vi "Test-Streaming.vi"() -> ()   [LabVIEW 2020]
uses:
  g_industrial_cam/Camera/Camera.lvclass
  g_industrial_cam/Buffer/Buffer.lvclass
  <vilib>/picture/picture.llb/Draw 8-Bit Pixmap.vi
  g_industrial_cam/Device Enumeration.ctl
panel:
  out "Trigger Source":string
  out "Streaming":bool
  out "Stream Restart Error":errorcluster
  in  "Stop Stream":bool
  in  "Start Stream":bool
  out "Timeout":bool
  out "Devices":T1[](array[typedef])
  in  "Picture Zoom Factor":sgl
  out "2D Picture":picture
  out "Snap Shot Count":i32
  in  "stop":bool
  out "error out":errorcluster
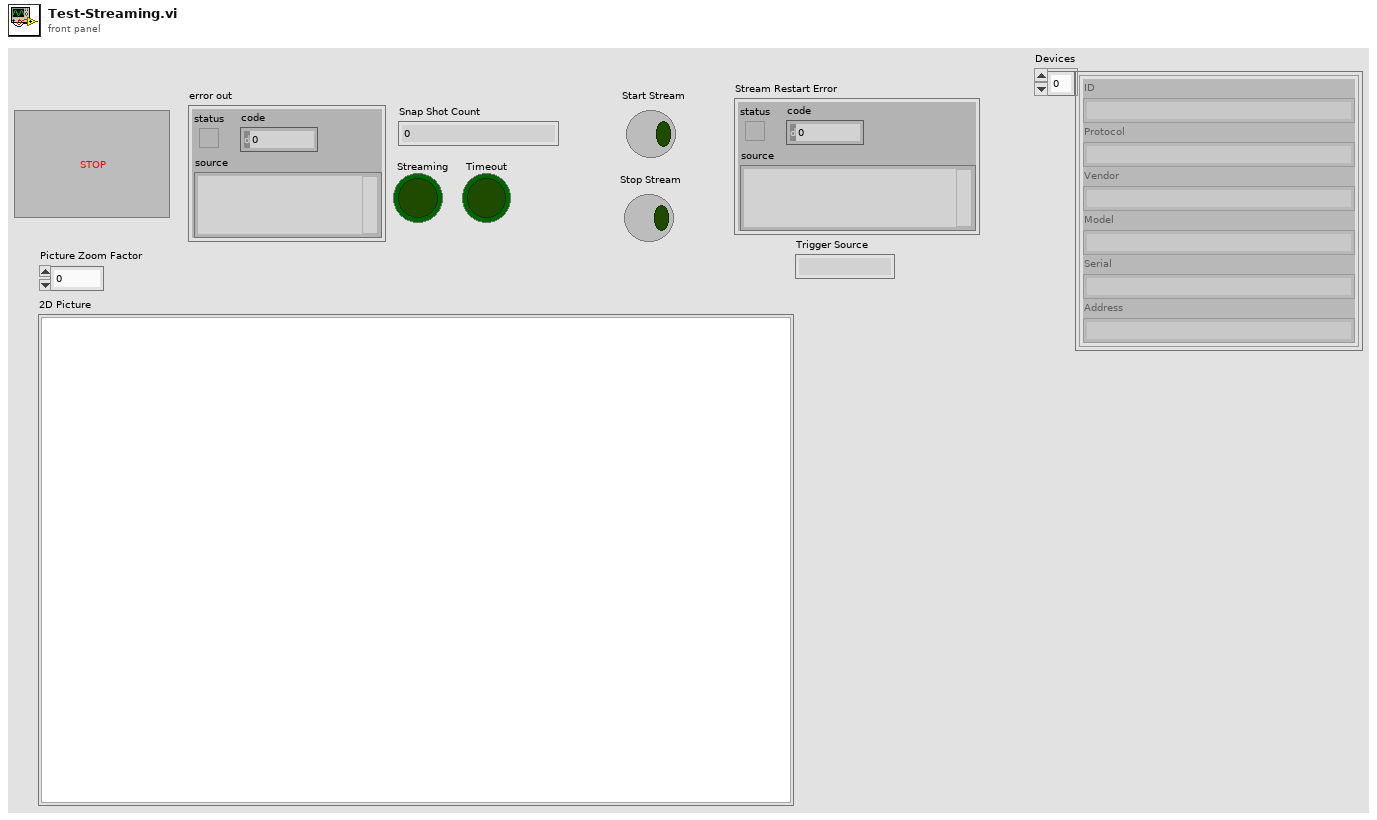
[diagram p1: front panel]
types:
  T1 = typedef "Device Enumeration.ctl" = cluster{"ID":string, "Protocol":string, "Vendor":string, "Model":string, "Serial":string, "Address":string}
  T2 = typedef "Buffer.lvclass/Image Size.ctl" = cluster{"Width":u16, "Height":u16}
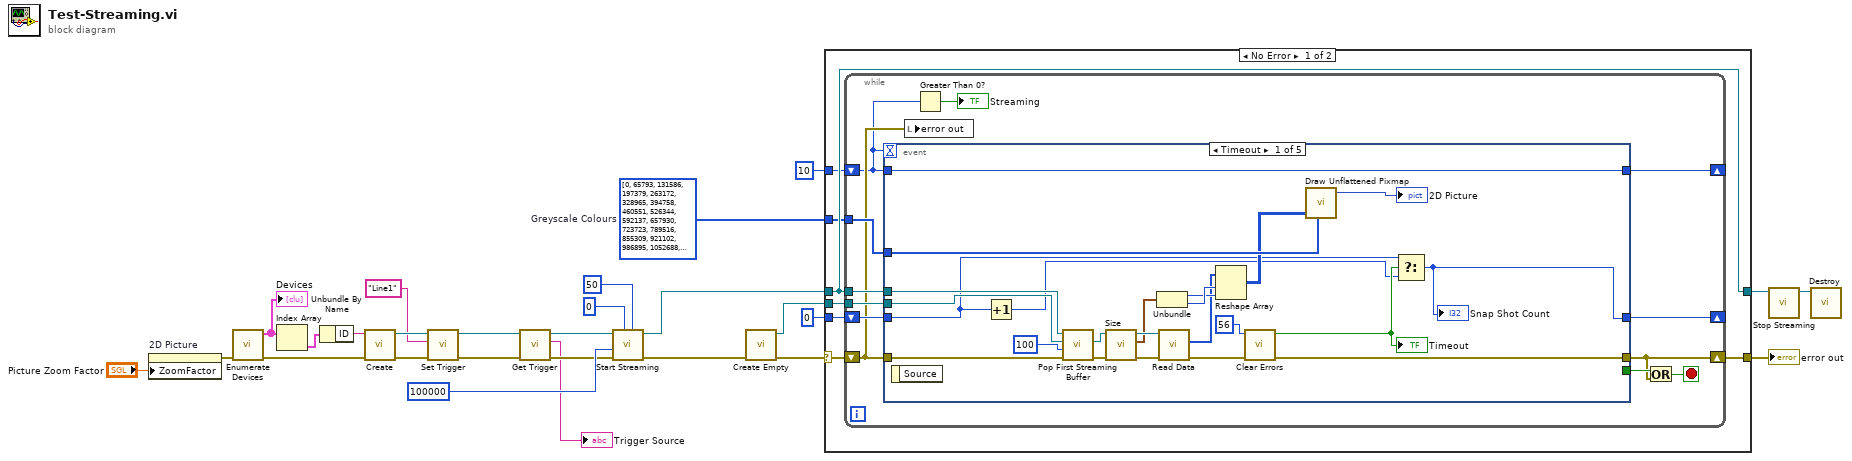
[diagram p0: block diagram]
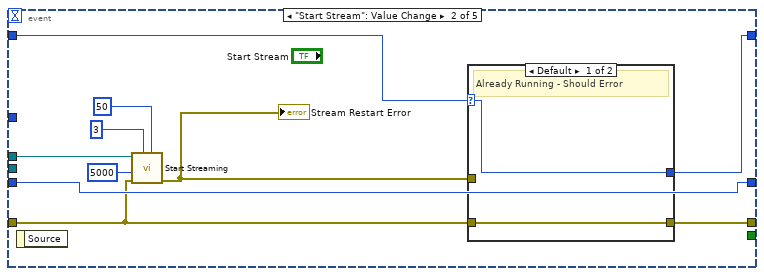
[diagram p2: hidden frame]
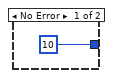
[diagram p4: hidden frame]
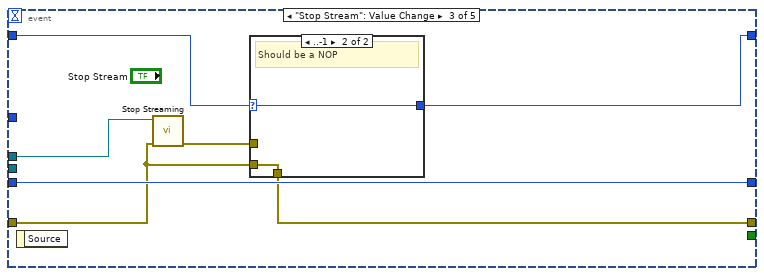
[diagram p5: hidden frame]
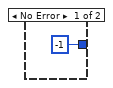
[diagram p7: hidden frame]
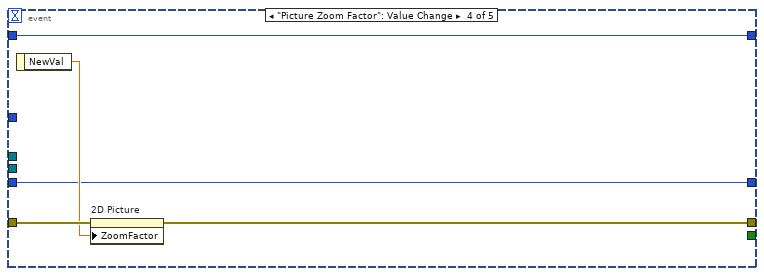
[diagram p8: hidden frame]
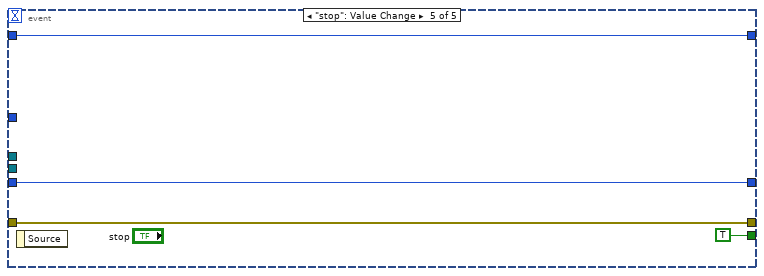
[diagram p9: hidden frame]
diagram:
  w21 = u32[] [0, 65793, 131586, 197379, 263172, 328965, 394758, 460551, 526344, 592137, 657930, 723723, 789516, 855309, 921102, 986895, 1052688, 1118481, 1184274, 1250067, 1315860, 1381653, 1447446, 1513239, 1579032, 1644825, 1710618, 1776411, 1842204, 1907997, 1973790, 2039583, 2105376, 2171169, 2236962, 2302755, 2368548, 2434341, 2500134, 2565927, 2631720, 2697513, 2763306, 2829099, 2894892, 2960685, 3026478, 3092271, 3158064, 3223857, 3289650, 3355443, 3421236, 3487029, 3552822, 3618615, 3684408, 3750201, 3815994, 3881787, 3947580, 4013373, 4079166, 4144959, 4210752, 4276545, 4342338, 4408131, 4473924, 4539717, 4605510, 4671303, 4737096, 4802889, 4868682, 4934475, 5000268, 5066061, 5131854, 5197647, 5263440, 5329233, 5395026, 5460819, 5526612, 5592405, 5658198, 5723991, 5789784, 5855577, 5921370, 5987163, 6052956, 6118749, 6184542, 6250335, 6316128, 6381921, 6447714, 6513507, 6579300, 6645093, 6710886, 6776679, 6842472, 6908265, 6974058, 7039851, 7105644, 7171437, 7237230, 7303023, 7368816, 7434609, 7500402, 7566195, 7631988, 7697781, 7763574, 7829367, 7895160, 7960953, 8026746, 8092539, 8158332, 8224125, 8289918, 8355711, 8421504, 8487297, 8553090, 8618883, 8684676, 8750469, 8816262, 8882055, 8947848, 9013641, 9079434, 9145227, 9211020, 9276813, 9342606, 9408399, 9474192, 9539985, 9605778, 9671571, 9737364, 9803157, 9868950, 9934743, 10000536, 10066329, 10132122, 10197915, 10263708, 10329501, 10395294, 10461087, 10526880, 10592673, 10658466, 10724259, 10790052, 10855845, 10921638, 10987431, 11053224, 11119017, 11184810, 11250603, 11316396, 11382189, 11447982, 11513775, 11579568, 11645361, 11711154, 11776947, 11842740, 11908533, 11974326, 12040119, 12105912, 12171705, 12237498, 12303291, 12369084, 12434877, 12500670, 12566463, 12632256, 12698049, 12763842, 12829635, 12895428, 12961221, 13027014, 13092807, 13158600, 13224393, 13290186, 13355979, 13421772, 13487565, 13553358, 13619151, 13684944, 13750737, 13816530, 13882323, 13948116, 14013909, 14079702, 14145495, 14211288, 14277081, 14342874, 14408667, 14474460, 14540253, 14606046, 14671839, 14737632, 14803425, 14869218, 14935011, 15000804, 15066597, 15132390, 15198183, 15263976, 15329769, 15395562, 15461355, 15527148, 15592941, 15658734, 15724527, 15790320, 15856113, 15921906, 15987699, 16053492, 16119285, 16185078, 16250871, 16316664, 16382457, 16448250, 16514043, 16579836, 16645629, 16711422, 16777215]  # Greyscale Colours
  n1 = property on="2D Picture" class="Pict"("ZoomFactor"="Picture Zoom Factor") -> (error out=w20:errorcluster)  [unwired: 2 in, 1 out]
  n2 = call "Enumerate Devices.vi"("error in (no error)"=w20) -> ("error out"=w25:errorcluster, "Devices"=w27:T1[])  [unwired: 9 in]
  "Devices" <- w27
  n3 = Index Array(array=w27) -> (element=w26:T1)  [unwired: 1 in]
  n4 = Unbundle By Name(w26) -> ("ID"=w24:string)
  n5 = call "Create.vi"("error in (no error)"=w25, "Identifier (ID, IP etc)"=w24) -> ("error out"=w23:errorcluster, "Camera"=w6:refnum<class "Camera.lvclass">)  [unwired: 8 in]
  n6 = call "Set Trigger.vi"("error in (no error)"=w23, "Source"="Line1", "Camera in"=w6) -> ("error out"=w7:errorcluster, "Camera"=w3:refnum<class "Camera.lvclass">)  [unwired: 7 in]
  n7 = call "Get Trigger.vi"("error in (no error)"=w7, "Camera in"=w3) -> ("error out"=w4:errorcluster, "Trigger Source"=→"Trigger Source":string, "Camera"=w2:refnum<class "Camera.lvclass">)  [unwired: 7 in]
  n8 = call "Start Streaming.vi"("Max Sequential Frame-Errors (Default: -1)"=50 ("Max Sequential Errors (Default: -1)"), "Additional Buffers (Default: 3)"=u16 0 ("Additional Buffers (3)"), "error in (no error)"=w4, "Timeout (ms)"=100000, "Camera in"=w2) -> ("error out"=w17:errorcluster, "Camera"=w18:refnum<class "Camera.lvclass">)  [unwired: 5 in]
  n9 = call "Create Empty.vi"("error in (no error)"=w17) -> ("error out"=w16:errorcluster, "Buffer out"=w15:refnum<class "Buffer.lvclass">)  [unwired: 9 in]
  n10 = case shown="No Error" w16 {
    selector: w16 -> [w34 w110]
    tunnel: w18 -> [w32 w111]
    tunnel: [w33 w110] -> w9
    tunnel: [w32 w111] -> w22
    tunnel: w21 -> [w31 _]
    tunnel: w15 -> [w30 _]
    tunnel: 0 -> [w29 _]
    tunnel: 10 -> [w28 _]
    frame No Error {
      n11 = while {
        shift-right: [w39] -> w33
        shift-left: w34 -> [w38]
        tunnel: w32 -> [w46]
        tunnel: w31 -> [w43]
        tunnel: w30 -> [w42]
        shift-right: [w40] -> _
        shift-left: w29 -> [w41]
        shift-right: [w37] -> _
        shift-left: w28 -> [w36]
        stop <- w44 stop-if-true
        n12 = event shown="[0] Timeout" {
          selector: _ -> [_ _ _ _ _]
          dyn-events: _ -> [_ _ _ _ _]
          timeout: w36 -> [_ _ _ _ _]
          tunnel: w46 -> [w69 w78 w92 _ _]
          tunnel: w38 -> [w68 w70 w87 w105 w109]
          tunnel: [w67 w71 w88 w104 w109] -> w39
          tunnel: [_ _ _ _ TRUE] -> w45
          tunnel: w43 -> [w66 _ _ _ _]
          tunnel: w42 -> [w64 _ _ _ _]
          tunnel: w41 -> [w49 w79 w93 w102 w107]
          tunnel: [w48 w79 w93 w102 w107] -> w40
          tunnel: [w47 w72 w89 w101 w106] -> w37
          tunnel: w36 -> [w47 w74 w91 w101 w106]
          event Timeout {
            n13 = event-data() -> ()  [unwired: 1 in, 1 out]
            n14 = Increment(x=w49) -> (x+1=w50:i32)
            n15 = call "Pop First Streaming Buffer.vi"("error in (no error)"=w68, "Timeout (ms) Default: -1"=100, "Buffer in"=w64, "Camera in"=w69) -> ("error out"=w62:errorcluster, "Buffer"=w63:refnum<class "Buffer.lvclass">)  [unwired: 5 in, 1 out]
            n16 = call "Size.vi"("error in (no error)"=w62, "Buffer Data in"=w63) -> ("error out"=w61:errorcluster, "Image Size"=w59:T2, "Buffer Data"=w60:refnum<class "Buffer.lvclass">)  [unwired: 7 in]
            n17 = Unbundle(w59) -> ("Width"=w57:u16, "Height"=w58:u16)
            n18 = call "Read Data.vi"("error in (no error)"=w61, "Buffer in"=w60) -> ("error out"=w56:errorcluster, "Data"=w55:u8[])  [unwired: 7 in, 1 out]
            n19 = Reshape Array(w55, w58, w57) -> (w54:u8[][])
            n20 = call <vilib>:"Clear Errors.vi"("error in (no error)"=w56, "specific error code to clear (0: all)"=56) -> ("error out"=w67:errorcluster, "specific error cleared?"=w51:bool)  [unwired: 4 in]
            "Timeout" <- w51
            n21 = call-poly <vilib>:"Draw Unflattened Pixmap.vi"("data"=w54, "color table"=w66) -> ("new picture"=→"2D Picture":picture)  [unwired: 7 in]
            n22 = Select(t=w49, s=w51, f=w50) -> (s? t:f=w48:i32)
            "Snap Shot Count" <- w48
          }
          event "Start Stream": Value Change {
            n23 = event-data() -> ()  [unwired: 1 in, 1 out]
            n24 = call "Start Streaming.vi"("Max Sequential Frame-Errors (Default: -1)"=50 ("Max Sequential Errors (Default: -1)"), "Additional Buffers (Default: 3)"=u16 3, "error in (no error)"=w70, "Timeout (ms)"=5000, "Camera in"=w78) -> ("error out"=w73:errorcluster)  [unwired: 5 in, 1 out]
            "Stream Restart Error" <- w73
            n25 = case shown="Default" w74 {
              selector: w74 -> [w81 w83]
              tunnel: w73 -> [_ w82]
              tunnel: [w81 w84] -> w72
              tunnel: [w80 w82] -> w71
              tunnel: w70 -> [w80 _]
              frame Default {
                # "Already Running - Should Error"
              }
              frame ..-1 {
                # "Should Have Started OK"
                n26 = case shown="Error .." w82 {
                  tunnel: [10 w86] -> w84
                  tunnel: w83 -> [_ w86]
                  frame No Error {
                  }
                  frame Error {
                  }
                }
              }
            }
          }
          event "Stop Stream": Value Change {
            n27 = event-data() -> ()  [unwired: 1 in, 1 out]
            n28 = call "Stop Streaming.vi"("error in (no error)"=w87, "Camera in"=w92) -> ("error out"=w90:errorcluster)  [unwired: 8 in, 1 out]
            n29 = case shown="..-1" w91 {
              selector: w91 -> [w95 w99]
              tunnel: w90 -> [w94 _]
              tunnel: [w96 w99] -> w89
              tunnel: [w94 w100] -> w88
              tunnel: w87 -> [_ w100]
              frame Default {
                # "Should Stop"
                n30 = case shown="Error .." w94 {
                  tunnel: [-1 w98] -> w96
                  tunnel: w95 -> [_ w98]
                  frame No Error {
                  }
                  frame Error {
                  }
                }
              }
              frame ..-1 {
                # "Should be a NOP"
              }
            }
          }
          event "Picture Zoom Factor": Value Change {
            n31 = event-data() -> ("NewVal"=w103:sgl)  [unwired: 1 in]
            n32 = property on="2D Picture" class="Pict"(error in=w105, "ZoomFactor"=w103) -> (error out=w104:errorcluster)  [unwired: 1 in, 1 out]
          }
          event "stop": Value Change {
            n33 = event-data() -> ()  [unwired: 1 in, 1 out]
          }
        }
        n34 = local write "error out"(w38) -> ()
        n35 = Greater Than 0?(x=w36) -> (x > 0?=→"Streaming":bool)
        n36 = Or(x=w45, y=w39) -> (x .or. y?=w44:bool)
      }
    }
    frame Error {
    }
  }
  "error out" <- w9
  n37 = call "Stop Streaming.vi"("Camera in"=w22) -> ("Camera"=w12:refnum<class "Camera.lvclass">)  [unwired: 9 in, 1 out]
  n38 = call "Destroy.vi"("Camera in"=w12) -> ()  [unwired: 10 in, 1 out]
